vi "Get Cal Coeffs.vi"(0 "DAQ Rack Number":u32, 5 "Cal Files Path":path, 7 "System Type":T1=enum."Deformation", 11 "Error IN":errorcluster) -> (4 "AI Coeffs":cluster{"Coefficients":dbl[]}[](array[cluster]), 15 "Error OUT":errorcluster)   [LabVIEW 2023]
uses:
  Type Defs and Controls/System Type.ctl
  <vilib>/Utility/file.llb/Read From Spreadsheet File (string).vi
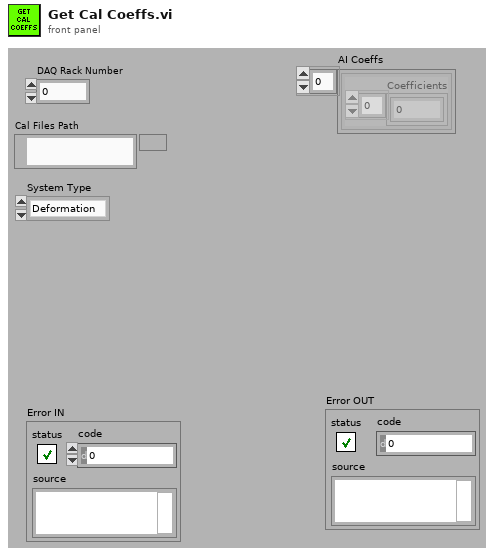
[diagram p1: front panel]
types:
  T1 = typedef "System Type.ctl" = enum16{"Standard", "Deformation", "Standard 8TC"}
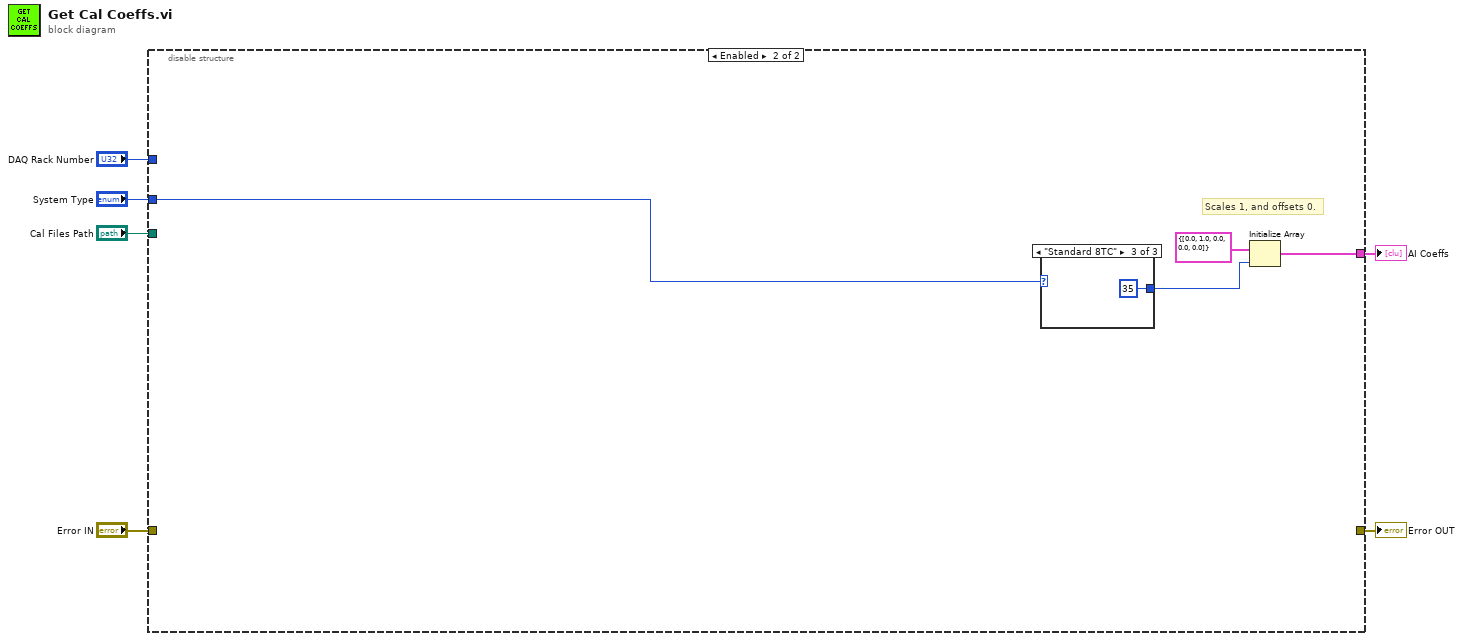
[diagram p0: block diagram]
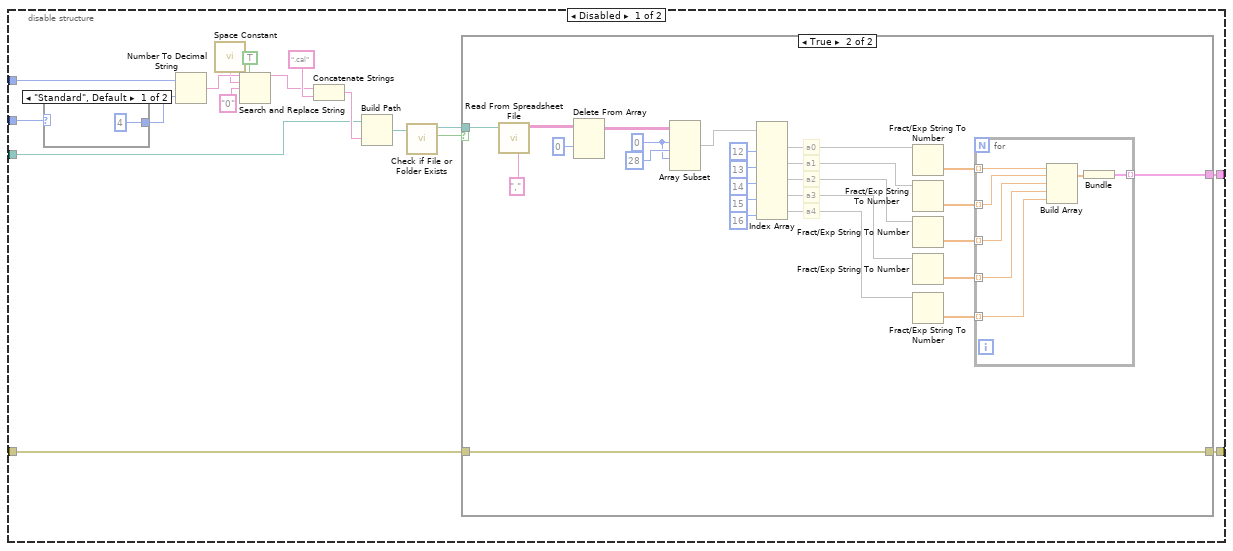
[diagram p2: hidden frame]
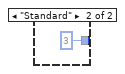
[diagram p3: hidden frame]
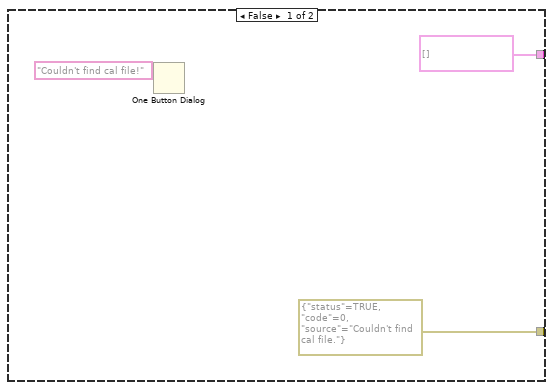
[diagram p4: hidden frame]
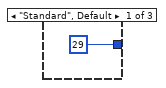
[diagram p5: hidden frame]
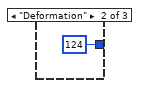
[diagram p6: hidden frame]
diagram:
  n1 = disable-structure shown="Enabled" {
    disable-tunnel: "DAQ Rack Number" -> [w18 _]
    disable-tunnel: [w17 w61] -> w5
    disable-tunnel: "Error IN" -> [w16 _]
    disable-tunnel: [w15 _] -> w3
    disable-tunnel: "Cal Files Path" -> [w9 _]
    disable-tunnel: "System Type" -> [w8 w63]
    frame Disabled {
      n2 = case shown="\"Standard\", Default" w8 {
        tunnel: [i16 4 ("width (-)") i16 3 ("width (-)")] -> w7
        frame "Standard", Default {
        }
        frame "Standard" {
        }
      }
      n3 = Number To Decimal String(number=w18, width (-)=w7) -> (decimal integer string=w14:string)
      n4 = call <vilib>:"Space Constant.vi"() -> ("String"=w13:string)
      n5 = Search and Replace String(replace all?=TRUE ("replace all? (F)"), input string=w14, search string=w13, replace string="0" ("replace string (\"\")")) -> (result string=w11:string)  [unwired: 4 in, 3 out]
      n6 = Concatenate Strings(w11, ".cal" ("string")) -> (w20:string)
      n7 = Build Path(base path=w9, name or relative path=w20) -> (appended path=w23:path)
      n8 = call <vilib>:"Check if File or Folder Exists.vi"("path"=w23) -> ("file or folder exists?"=w22:bool, "dup path"=w21:path)  [unwired: 8 in, 1 out]
      n9 = case shown="True" w22 {
        tunnel: w21 -> [_ w53]
        tunnel: [cluster{dbl[]}[] [] w35] -> w17
        tunnel: [errorcluster {"status"=TRUE, "code"=0, "source"="Couldn't find cal file."} ("error out") w38] -> w15
        tunnel: w16 -> [_ w38]
        frame False {
          n10 = One Button Dialog(message="Couldn't find cal file!") -> ()  [unwired: 1 in, 1 out]
        }
        frame True {
          w47 = 0 ("index")
          # "a4"
          # "a3"
          # "a2"
          # "a1"
          # "a0"
          n11 = call-poly <vilib>:"Read From Spreadsheet File.vi"("delimiter (\\t)"="," ("delimiter (\\t)"), "file path (dialog if empty)"=w53) -> ("all rows"=w52:string[][])  [unwired: 5 in, 4 out]
          n12 = Delete From Array(array=w52, index (row)=0) -> (array with subset deleted=w36:string[][])  [unwired: 2 in, 1 out]
          n13 = Array Subset(array=w36, index (row)=w47, length (row)=28 ("length"), index (col)=w47) -> (w37:string[][])  [unwired: 1 in]
          n14 = Index Array(array=w37, index (col) #1=12 ("disabled index (col)"), index (col) #2=13 ("disabled index (col)"), index (col) #3=14 ("disabled index (col)"), index (col) #4=15 ("disabled index (col)"), index (col) #5=16 ("disabled index (col)")) -> (element #1=w46:string[], element #2=w45:string[], element #3=w42:string[], element #4=w34:string[], element #5=w33:string[])  [unwired: 5 in]
          n15 = Fract/Exp String To Number(string=w46) -> (number=w41:dbl[])  [unwired: 3 in, 1 out]
          n16 = Fract/Exp String To Number(string=w45) -> (number=w40:dbl[])  [unwired: 3 in, 1 out]
          n17 = Fract/Exp String To Number(string=w42) -> (number=w39:dbl[])  [unwired: 3 in, 1 out]
          n18 = Fract/Exp String To Number(string=w34) -> (number=w30:dbl[])  [unwired: 3 in, 1 out]
          n19 = Fract/Exp String To Number(string=w33) -> (number=w29:dbl[])  [unwired: 3 in, 1 out]
          n20 = for {
            tunnel: w41 -> [w60] mode=indexing
            tunnel: w40 -> [w59] mode=indexing
            tunnel: w39 -> [w58] mode=indexing
            tunnel: [w56] -> w35 mode=indexing
            tunnel: w30 -> [w55] mode=indexing
            tunnel: w29 -> [w54] mode=indexing
            n21 = Build Array(w60, w59, w58, w55, w54) -> (w57:dbl[])
            n22 = Bundle(w57) -> (w56:cluster{dbl[]})  [unwired: 1 in]
          }
        }
      }
    }
    frame Enabled {
      # "Scales 1, and offsets 0."
      n23 = case shown="\"Standard 8TC\"" w63 {
        tunnel: [29 ("dimension size") 124 ("dimension size") 35 ("dimension size")] -> w62
        frame "Standard", Default {
        }
        frame "Deformation" {
        }
        frame "Standard 8TC" {
        }
      }
      n24 = Initialize Array(cluster{dbl[]} {[0.0, 1.0, 0.0, 0.0, 0.0]}, w62) -> (w61:cluster{dbl[]}[])
    }
  }
  "AI Coeffs" <- w5
  "Error OUT" <- w3
